vi "Tool Q LEIN controller relay complex task.vi"(0 "Controller ID":u8=42, 1 "Relay 1 close(on)":bool, 5 "current limit(0.2A)":dbl, 9 "time (50 ms)":u16=50, 11 "error in (no error)":errorcluster, 12 "Relay 2 close(on)":bool) -> (4 "LEIN custom reply Q":T1, 15 "error out":errorcluster)   [LabVIEW 2011]
uses:
  LEINmaster/Defenitions/LEIN custom reply Q.ctl
  LEINmaster/Defenitions/LEIN Reply Holder.ctl
  LEINmaster/Defenitions/LEIN CMD Cluster.ctl
  LEINmaster/Defenitions/LEIN CMD List.ctl
  LEINmaster/Defenitions/LEIN Structure variations.ctl
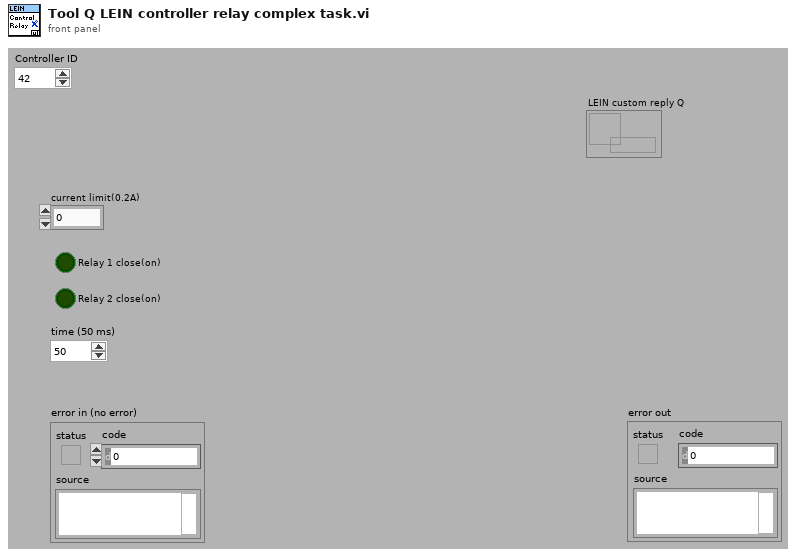
[diagram p1: front panel]
types:
  T1 = typedef "LEIN custom reply Q.ctl" = refnum<queue>
  T2 = typedef "LEIN Structure variations.ctl" = enum16{"LEIN08", "LEIN31", "LEIN63"}
  T3 = enum16{"big-endian, network order", "native, host order", "little-endian"}
  T4 = typedef "LEIN CMD Cluster.ctl" = cluster{"SID":u8, "ANF":bool, "CMD":T5, "DATA":u8[]}
  T5 = typedef "LEIN CMD List.ctl" = enum8{"ACTI", "TASK", "RES0", "STAT", "RES1", "RES2", "RES3", "USER"}
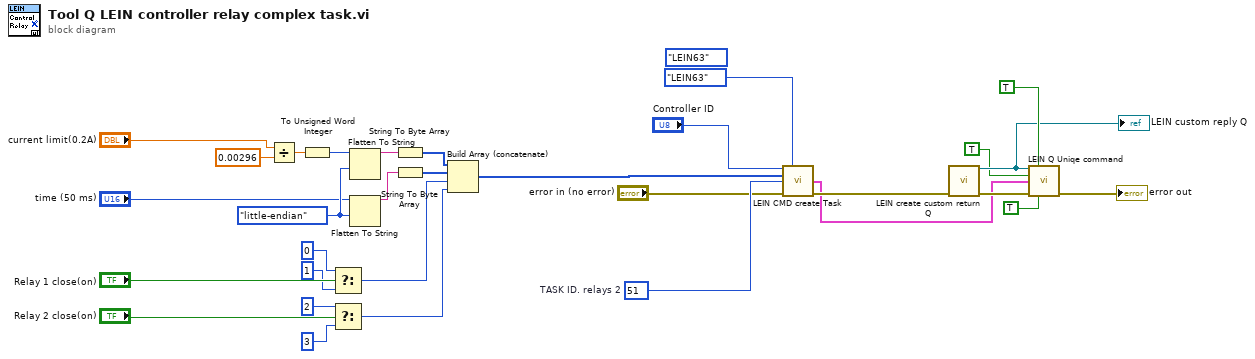
[diagram p0: block diagram]
diagram:
  (unwired) LEIN_Structure_variations."LEIN63" ("LEIN Variation")
  w20 = u8 51  # TASK ID. relays 2
  w25 = T3."little-endian" ("byte order (0:big-endian, network order)")
  n1 = Divide(x="current limit(0.2A)", y=0.00296 ("x")) -> (x/y=w30:dbl)
  n2 = To Unsigned Word Integer(number=w30) -> (unsigned 16bit integer=w28:u16)
  n3 = Select(t=u8 0 ("outpuyt channel"), s="Relay 1 close(on)", f=u8 1 ("outpuyt channel")) -> (s? t:f=w8:u8)
  n4 = Select(t=u8 2 ("outpuyt channel"), s="Relay 2 close(on)", f=u8 3 ("outpuyt channel")) -> (s? t:f=w7:u8)
  n5 = Flatten To String(anything=w28, byte order (0:big-endian, network order)=w25) -> (data string=w27:string)  [unwired: 2 in, 2 out]
  n6 = Flatten To String(anything="time (50 ms)", byte order (0:big-endian, network order)=w25) -> (data string=w23:string)  [unwired: 2 in, 2 out]
  n7 = String To Byte Array(string=w27) -> (unsigned byte array=w26:u8[])
  n8 = String To Byte Array(string=w23) -> (unsigned byte array=w22:u8[])
  n9 = Build Array (concatenate)(w26, w22, w8, w7) -> (w18:u8[])
  n10 = call "LEIN CMD create Task.vi"("SID"="Controller ID", "LEIN Variation"=LEIN_Structure_variations."LEIN63", "Data"=w18, "TASK ID"=w20, "error in (no error)"="error in (no error)") -> ("CMD"=w1:T4, "error out"=w5:errorcluster)  [unwired: 9 in]
  n11 = call "LEIN create custom return Q.vi"("error in (no error)"=w5) -> ("LEIN custom reply Q"=w3:T1, "error out"=w4:errorcluster)  [unwired: 13 in]
  "LEIN custom reply Q" <- w3
  n12 = call "LEIN Q Uniqe command.vi"("LEIN custom reply Q"=w3, "Retry on err (F)"=TRUE, "Custom Q(F)"=TRUE, "CMD"=w1, "error in"=w4, "priority(F)"=TRUE) -> ("error out"=→"error out":errorcluster)  [unwired: 9 in]
